vi "Get Assertion Message From Test Case.vi"(8 "error in (no error)":errorcluster, 11 "Test Case Test Double in":refnum<class "Test Case Test Double.lvclass">) -> (0 "error out":errorcluster, 3 "Message":string)   [LabVIEW 2020, in "LUnit Tests.lvlib" / "Assertion Result Test.lvclass"]
uses:
  Assertion Result Test.lvclass
  Test Dummys/Test Case Test Double/Test Case Test Double.lvclass
  C:/Git/astemes-lunit/source/Framework/Test Case/LUnit Test Case.lvclass
  source/Framework/Test Case/LUnit Test Case.lvclass/LUnit Test Case.ctl
  source/Framework/Test Case/LUnit Test Case.lvclass
  source/Framework/Result Types/Case Result/Test Case Result.lvlib
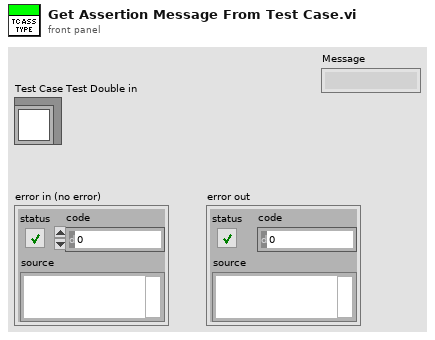
[diagram p1: front panel]
types:
  T1 = typedef "Test Case Result.lvlib/Test Case Result type.ctl" = map{string, T2}
  T2 = typedef "Method Result.lvlib/Method Result type.ctl" = cluster{"Test Case":string, "Test Method Name":string, "Status":T3, "Assertion Results":T4[], "Execution time":dbl, "Result String":string}
  T3 = typedef "Assertion Result.lvlib/Status.ctl" = enum16{"Pass", "Fail", "Error", "Skipped", "Setup Error", "Broken", "Teardown Error"}
  T4 = typedef "Assertion Result.lvlib/Assertion Result type.ctl" = cluster{"Status":T3, "Message":string, "Description":string, "Assertion Type":T5}
  T5 = typedef "Assertion Result.lvlib/Assertion Type.ctl" = enum16{"None", "Pass", "Fail", "Skip", "Pass if Equal", "Fail if Equal", "Pass if Error", "Fail if Error", "Pass if", "Fail if"}
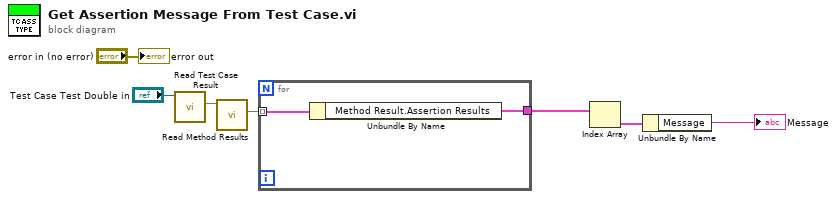
[diagram p0: block diagram]
diagram:
  n1 = call "Read Test Case Result.vi"("LUnit Test Case In"="Test Case Test Double in") -> ("Test Case Result"=w6:T1)  [unwired: 9 in, 1 out]
  n2 = call "Read Method Results.vi"("Test Case Result In"=w6) -> ("Method Results"=w7:map{string, T2})  [unwired: 9 in, 1 out]
  n3 = for {
    tunnel: [w8] -> w1
    tunnel: w7 -> [w9] mode=indexing
    n4 = Unbundle By Name(w9) -> ("Method Result.Assertion Results"=w8:T4[])
  }
  n5 = Index Array(array=w1) -> (element=w3:T4)  [unwired: 1 in]
  n6 = Unbundle By Name(w3) -> ("Message"=→"Message":string)
  "error out" <- "error in (no error)"
